vi "Clear.vi"(8 "error in":errorcluster, 11 "Main Data Buffer In":T1) -> (0 "error out":errorcluster, 3 "Main Data Buffer Out":T1)   [LabVIEW 2020, in "SECS Bridge.lvlib"]
uses:
  SECS Bridge.lvlib
  Main Data Buffer.ctl
  SECS Communication/HSMS Class/HSMS Class.lvclass
  SECS Communication/SECS Data Class/SECS Data Class.lvclass
  SECS Scenarios/Scenarios Class/Scenarios Class.lvclass
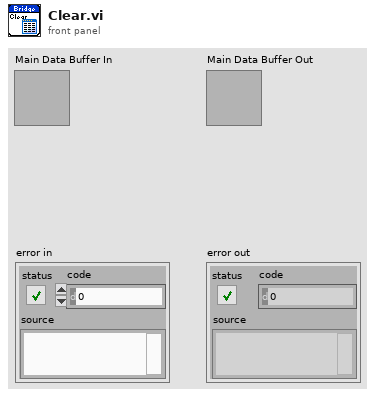
[diagram p1: front panel]
types:
  T1 = typedef "SECS Bridge.lvlib/Main Data Buffer.ctl" = cluster{"HSMS Class":refnum<class "HSMS Class.lvclass">, "SECS Data Class":refnum<class "SECS Data Class.lvclass">, "Scenarios Class":refnum<class "Scenarios Class.lvclass">, "VI Refnum":refnum<vi>, "Ctl Refnum Map":map{string, refnum<vi>}, "Timeout":i32, "Notifier Data":string[], "Event Refnum":refnum<event-registration>}
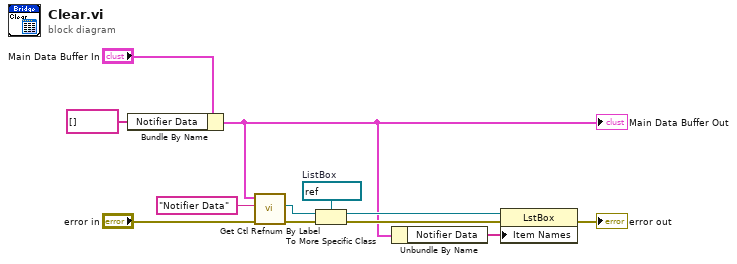
[diagram p0: block diagram]
diagram:
  w9 = refnum<vi> refnum  # ListBox
  n1 = Bundle By Name(cluster="Main Data Buffer In", "Notifier Data"=string[] []) -> (w2:T1)
  "Main Data Buffer Out" <- w2
  n2 = call "Get Ctl Refnum By Label.vi"("error in"="error in", "Label"="Notifier Data", "Main Data Buffer In"=w2) -> ("error out"=w11:errorcluster, "Ctl Refnum"=w10:refnum<vi>)  [unwired: 6 in, 1 out]
  n3 = To More Specific Class(target class=w9, reference=w10, error in=w11) -> (specific class reference=w7:refnum<vi>, error out=w8:errorcluster)
  n4 = Unbundle By Name(w2) -> ("Notifier Data"=w6:string[])
  n5 = property class="LstBox"(reference=w7, error in=w8, "Item Names"=w6) -> (error out=→"error out":errorcluster)  [unwired: 1 out]
